vi "LED Graph.vi"() -> ()   [LabVIEW 2020, in "CTI-Visa-Scratchpad.lvlib"]
uses:
  CTI-Visa-Scratchpad.lvlib
  CTI-Visa/CTI-Visa.lvlib
  CTI-Visa/Digital Direction.ctl
panel:
  out "Readback":bool[](array[boolean])
  in  "Port":refnum<visa-resource-name>="COM3"
  in  "stop":bool
  in  "Graph":u8(slide) scale=0.0..10.0
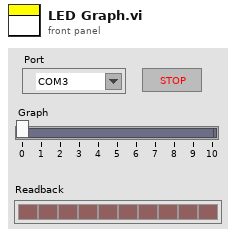
[diagram p1: front panel]
types:
  T1 = typedef "CTI-Visa.lvlib/Digital Direction.ctl" = enum16{"In", "Out"}
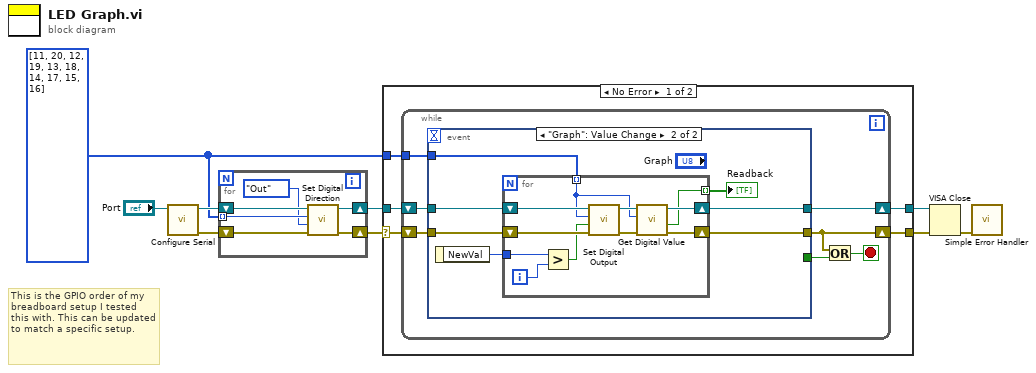
[diagram p0: block diagram]
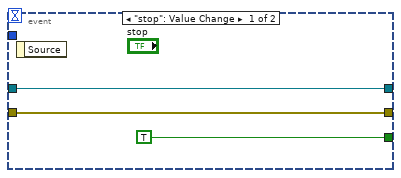
[diagram p2: hidden frame]
diagram:
  w4 = i32[] [11, 20, 12, 19, 13, 18, 14, 17, 15, 16]
  # "This is the GPIO order of my breadboard setup I tested this with. This can be updated to match a specific setup."
  n1 = call "Configure Serial.vi"("VISA resource name in"="Port") -> ("error out"=w7:errorcluster, "VISA resource name"=w8:refnum<visa-resource-name>)  [unwired: 9 in]
  n2 = for {
    tunnel: w4 -> [w14] mode=indexing
    shift-right: [w11] -> w5
    shift-left: w7 -> [w12]
    shift-right: [w10] -> w6
    shift-left: w8 -> [w15]
    n3 = call "Set Digital Direction.vi"("error in (no error)"=w12, "Direction"=Digital_Direction."Out", "Channel"=w14, "VISA resource name in"=w15) -> ("error out"=w11:errorcluster, "VISA resource name"=w10:refnum<visa-resource-name>)  [unwired: 6 in]
  }
  n4 = case shown="No Error" w5 {
    selector: w5 -> [w19 w49]
    tunnel: w6 -> [w20 w50]
    tunnel: w4 -> [w18 _]
    tunnel: [w17 w50] -> w3
    tunnel: [w16 w49] -> w2
    frame No Error {
      n5 = while {
        shift-right: [w25] -> w17
        shift-left: w20 -> [w27]
        shift-right: [w24] -> w16
        shift-left: w19 -> [w26]
        tunnel: w18 -> [w21]
        stop <- w23 stop-if-true
        n6 = event shown="[1] \"Graph\": Value Change" {
          selector: _ -> [_ _]
          dyn-events: _ -> [_ _]
          timeout: _ -> [_ _]
          tunnel: w27 -> [w30 w36]
          tunnel: w26 -> [w29 w35]
          tunnel: [w30 w33] -> w25
          tunnel: [w29 w32] -> w24
          tunnel: [TRUE _] -> w22
          tunnel: w21 -> [_ w34]
          event "stop": Value Change {
            n7 = event-data() -> ()  [unwired: 1 in, 1 out]
          }
          event "Graph": Value Change {
            n8 = event-data() -> ("NewVal"=w37:u8)  [unwired: 1 in]
            n9 = for {
              tunnel: w37 -> [w46]
              shift-right: [w40] -> w33
              shift-left: w36 -> [w48]
              shift-right: [w39] -> w32
              shift-left: w35 -> [w47]
              tunnel: w34 -> [w41] mode=indexing
              tunnel: [w38] -> w31 mode=indexing
              i -> [w45]
              n10 = Greater?(x=w46, y=w45) -> (0:w44:bool)
              n11 = call "Set Digital Output.vi"("error in (no error)"=w47, "Value"=w44, "Channel"=w41, "VISA resource name in"=w48) -> ("error out"=w42:errorcluster, "VISA resource name"=w43:refnum<visa-resource-name>)  [unwired: 6 in]
              n12 = call "Get Digital Value.vi"("error in (no error)"=w42, "Channel"=w41, "VISA resource name in"=w43) -> ("error out"=w39:errorcluster, "Value"=w38:bool, "VISA resource name"=w40:refnum<visa-resource-name>)  [unwired: 6 in]
            }
            "Readback" <- w31
          }
        }
        n13 = Or(x=w24, y=w22) -> (x .or. y?=w23:bool)
      }
    }
    frame Error {
    }
  }
  n14 = VISA Close(VISA resource name=w3, error in (no error)=w2) -> (error out=w1:errorcluster)
  n15 = call <vilib>:"Simple Error Handler.vi"("error in (no error)"=w1) -> ()  [unwired: 4 in, 5 out]
